vi "CleanupFileFolders.vi"(8 "error in (no error)":errorcluster) -> (0 "error out":errorcluster)   [LabVIEW 2017, in "FileManager.lvlib"]
uses:
  <vilib>/addons/InsightCM/Devices/Shared/Common/FileManager/FileManager.lvlib
  <vilib>/addons/InsightCM/Utilities/GlobalConfiguration/GlobalConfiguration.lvlib
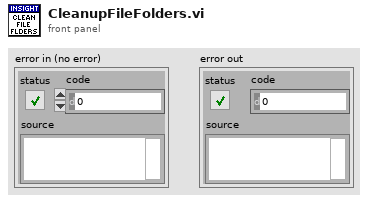
[diagram p1: front panel]
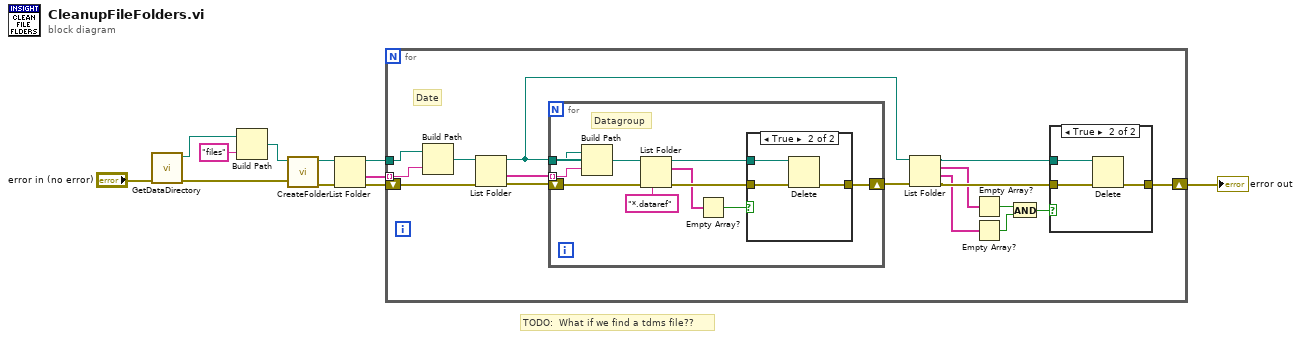
[diagram p0: block diagram]
diagram:
  # "TODO:  What if we find a tdms file??"
  n1 = call <vilib>:"GetDataDirectory.vi"("error in (no error)"="error in (no error)") -> ("error out"=w11:errorcluster, "data directory"=w10:path)  [unwired: 9 in]
  n2 = Build Path(base path=w10, name or relative path="files") -> (appended path=w6:path)
  n3 = call <vilib>:"CreateFolder.vi"("error in (no error)"=w11, "folder"=w6) -> ("error out"=w4:errorcluster, "folder out"=w5:path)  [unwired: 8 in]
  n4 = List Folder(path=w5, error in=w4) -> (path out=w7:path, folder names=w8:string[], error out=w9:errorcluster)  [unwired: 3 out]
  n5 = for {
    tunnel: w8 -> [w22] mode=indexing
    tunnel: w7 -> [w24]
    shift-right: [w16] -> w1
    shift-left: w9 -> [w27]
    # "Date"
    n6 = Build Path(base path=w24, name or relative path=w22) -> (appended path=w23:path)
    n7 = List Folder(path=w23, error in=w27) -> (path out=w20:path, folder names=w26:string[], error out=w25:errorcluster)  [unwired: 3 out]
    n8 = for {
      tunnel: w20 -> [w37]
      tunnel: w26 -> [w36] mode=indexing
      shift-right: [w35] -> w21
      shift-left: w25 -> [w28]
      # "Datagroup"
      n9 = Build Path(base path=w37, name or relative path=w36) -> (appended path=w30:path)
      n10 = List Folder(path=w30, pattern="*.dataref", error in=w28) -> (path out=w32:path, filenames=w31:string[], error out=w33:errorcluster)  [unwired: 2 out]
      n11 = Empty Array?(array=w31) -> (empty?=w29:bool)
      n12 = case shown="True" w29 {
        tunnel: w32 -> [_ w41]
        tunnel: w33 -> [w38 w40]
        tunnel: [w38 w39] -> w35
        frame False {
        }
        frame True {
          n13 = Delete(path (use dialog)=w41, error in=w40) -> (error out=w39:errorcluster)  [unwired: 3 in, 2 out]
        }
      }
    }
    n14 = List Folder(path=w20, error in=w21) -> (path out=w18:path, filenames=w14:string[], folder names=w15:string[], error out=w17:errorcluster)  [unwired: 2 out]
    n15 = Empty Array?(array=w14) -> (empty?=w13:bool)
    n16 = Empty Array?(array=w15) -> (empty?=w12:bool)
    n17 = And(x=w13, y=w12) -> (x .and. y?=w19:bool)
    n18 = case shown="True" w19 {
      tunnel: w18 -> [_ w45]
      tunnel: w17 -> [w42 w44]
      tunnel: [w42 w43] -> w16
      frame False {
      }
      frame True {
        n19 = Delete(path (use dialog)=w45, error in=w44) -> (error out=w43:errorcluster)  [unwired: 3 in, 2 out]
      }
    }
  }
  "error out" <- w1
